vi "Basic Pedestrian Lights.vi"() -> ()   [LabVIEW 2012]
doc: "VI which is to simply run through the traffic light routine whilst providing a pedestrian crossing system:\nRed -> RedAmber -> Green -> Amber -> Red (and check for boolean walk-button press)"
uses:
  Controls/Traffic Light Display.ctl
  Controls/Pedestrian Light Display.ctl
panel:
  out "Pedestrian Light Display":T1
  in  "Walk":bool
  in  "Stop Button":bool
  out "Traffic Light Display":T2
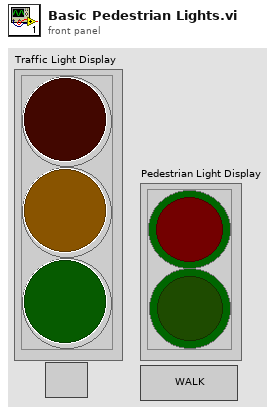
[diagram p1: front panel]
types:
  T1 = typedef "Pedestrian Light Display.ctl" = cluster{"Red":bool, "Green":bool}
  T2 = typedef "Traffic Light Display.ctl" = cluster{"RED":bool, "AMBER":bool, "GREEN":bool}
  T3 = enum16{"Red", "RedAmber", "Green", "Amber", "Walk"}
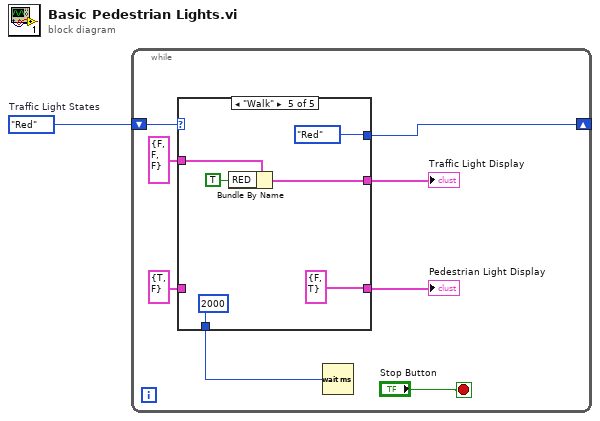
[diagram p0: block diagram]
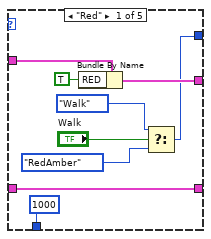
[diagram p2: hidden frame]
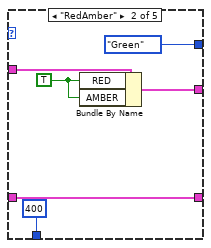
[diagram p3: hidden frame]
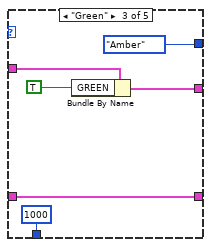
[diagram p4: hidden frame]
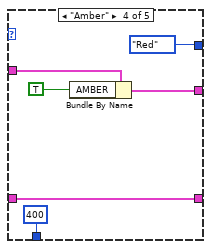
[diagram p5: hidden frame]
diagram:
  w1 = T3."Red"  # Traffic Light States
  n1 = while {
    shift-right: [w6] -> _
    shift-left: w1 -> [w9]
    stop <- "Stop Button" stop-if-true
    n2 = case shown="\"Walk\"" w9 {
      tunnel: T2 {"RED"=FALSE, "AMBER"=FALSE, "GREEN"=FALSE} ("Traffic Light Display") -> [w18 w24 w30 w36 w41]
      tunnel: [w16 w23 w28 w34 w39] -> w7
      tunnel: [w13 T3."Green" T3."Amber" T3."Red" T3."Red"] -> w6
      tunnel: [1000 400 1000 400 2000] -> w4
      tunnel: T1 {"Red"=TRUE, "Green"=FALSE} ("Pedestrian Light Display") -> [w12 w20 w26 w32 _]
      tunnel: [w12 w20 w26 w32 T1 {"Red"=FALSE, "Green"=TRUE} ("Pedestrian Light Display")] -> w2
      frame "Red" {
        n3 = Bundle By Name(cluster=w18, "RED"=TRUE) -> (w16:T2)
        n4 = Select(t=T3."Walk", s="Walk", f=T3."RedAmber") -> (s? t:f=w13:T3)
      }
      frame "RedAmber" {
        w22 = TRUE ("RED")
        n5 = Bundle By Name(cluster=w24, "RED"=w22, "AMBER"=w22) -> (w23:T2)
      }
      frame "Green" {
        n6 = Bundle By Name(cluster=w30, "GREEN"=TRUE ("RED")) -> (w28:T2)
      }
      frame "Amber" {
        n7 = Bundle By Name(cluster=w36, "AMBER"=TRUE ("RED")) -> (w34:T2)
      }
      frame "Walk" {
        n8 = Bundle By Name(cluster=w41, "RED"=TRUE) -> (w39:T2)
      }
    }
    "Traffic Light Display" <- w7
    "Pedestrian Light Display" <- w2
    n9 = Wait (ms)(milliseconds to wait=w4) -> ()  [unwired: 1 out]
  }
